vi "FGV_PSP - VRM Status.vi"(4 "error in":errorcluster, 6 "Function":enum16{"write", "read"}(ring), 7 "VRM status":T1={"X Target (T)"=0.0, "Y Target (T)"=0.0, "Z Target (T)"=0.0, "X Field (T)"=-0.0, "Y Field (T)"=0.0, "Z Field (T)"=0.0, "X Rate (T/min)"=0.0002, "Y Rate (T/min)"=0.0002, "Z Rate (T/min)"=0.05, "X Current (A)"=-0.0001, "Y Current (A)"=0.0001, "Z Current (A)"=0.0, "X Voltage (V)"=0.0003, "Y Voltage (V)"=0.0, "Z Voltage (V)"=-0.0001}) -> (0 "error out":errorcluster, 3 "VRM status":T1)   [LabVIEW 2016]
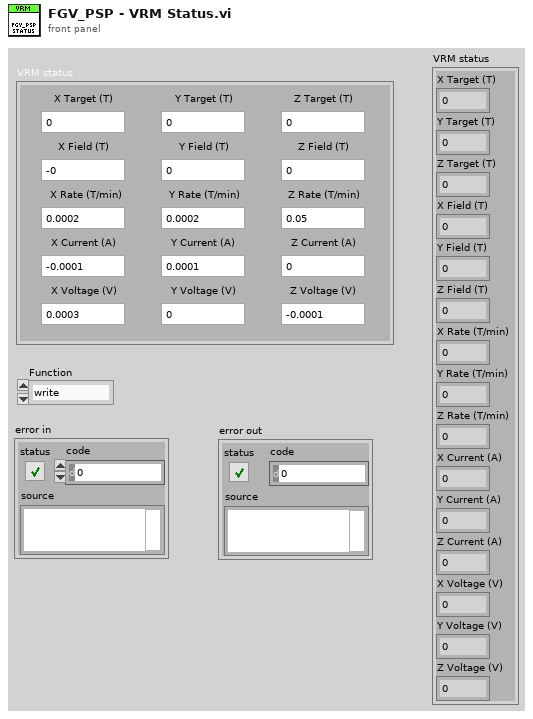
[diagram p1: front panel]
types:
  T1 = cluster{"X Target (T)":dbl, "Y Target (T)":dbl, "Z Target (T)":dbl, "X Field (T)":dbl, "Y Field (T)":dbl, "Z Field (T)":dbl, "X Rate (T/min)":dbl, "Y Rate (T/min)":dbl, "Z Rate (T/min)":dbl, "X Current (A)":dbl, "Y Current (A)":dbl, "Z Current (A)":dbl, "X Voltage (V)":dbl, "Y Voltage (V)":dbl, "Z Voltage (V)":dbl}
  T2 = cluster{"[0]":dbl, "[1]":dbl, "[2]":dbl, "[3]":dbl, "[4]":dbl, "[5]":dbl, "[6]":dbl, "[7]":dbl, "[8]":dbl, "[9]":dbl, "[10]":dbl, "[11]":dbl, "[12]":dbl, "[13]":dbl, "[14]":dbl}
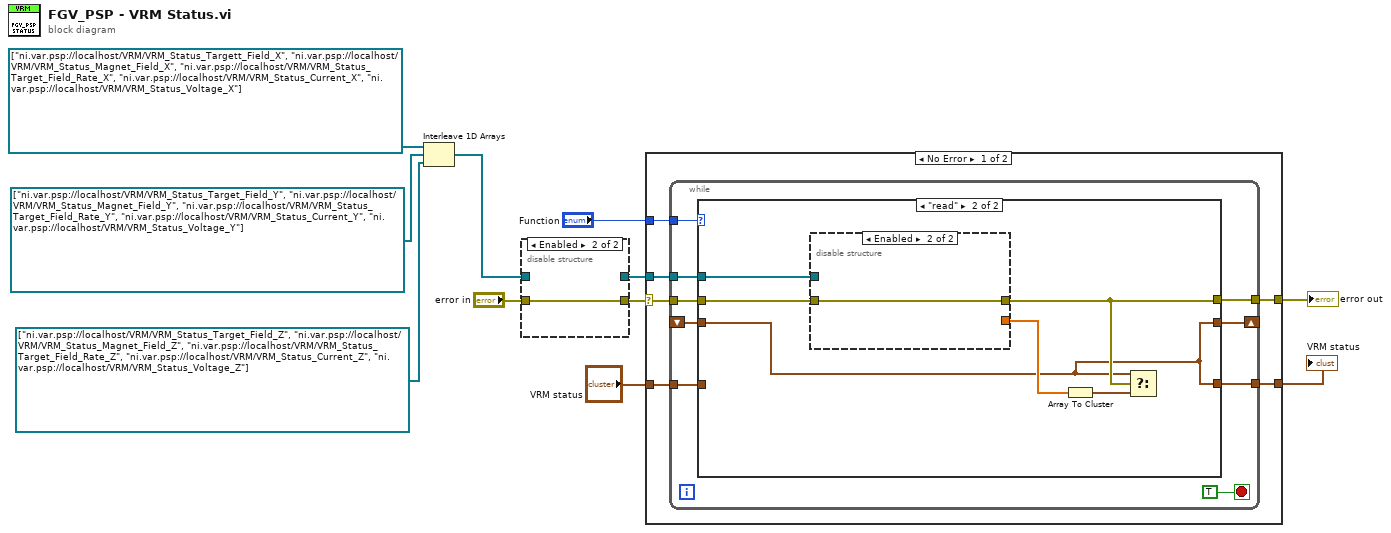
[diagram p0: block diagram]
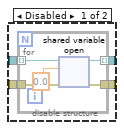
[diagram p2: hidden frame]
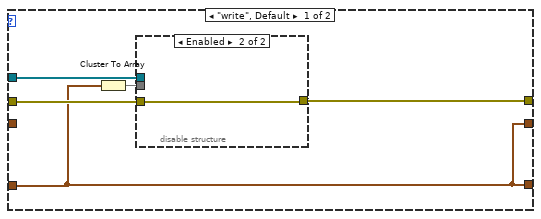
[diagram p3: hidden frame]
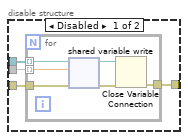
[diagram p4: hidden frame]
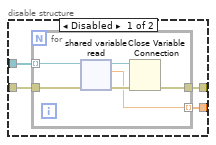
[diagram p5: hidden frame]
diagram:
  n1 = Interleave 1D Arrays(refnum<k21>[] ["ni.var.psp://localhost/VRM/VRM_Status_Targett_Field_X", "ni.var.psp://localhost/VRM/VRM_Status_Magnet_Field_X", "ni.var.psp://localhost/VRM/VRM_Status_Target_Field_Rate_X", "ni.var.psp://localhost/VRM/VRM_Status_Current_X", "ni.var.psp://localhost/VRM/VRM_Status_Voltage_X"], refnum<k21>[] ["ni.var.psp://localhost/VRM/VRM_Status_Target_Field_Y", "ni.var.psp://localhost/VRM/VRM_Status_Magnet_Field_Y", "ni.var.psp://localhost/VRM/VRM_Status_Target_Field_Rate_Y", "ni.var.psp://localhost/VRM/VRM_Status_Current_Y", "ni.var.psp://localhost/VRM/VRM_Status_Voltage_Y"], refnum<k21>[] ["ni.var.psp://localhost/VRM/VRM_Status_Target_Field_Z", "ni.var.psp://localhost/VRM/VRM_Status_Magnet_Field_Z", "ni.var.psp://localhost/VRM/VRM_Status_Target_Field_Rate_Z", "ni.var.psp://localhost/VRM/VRM_Status_Current_Z", "ni.var.psp://localhost/VRM/VRM_Status_Voltage_Z"]) -> (w1:refnum<k21>[])
  n2 = disable-structure shown="Enabled" {
    disable-tunnel: "error in" -> [w15 w21]
    disable-tunnel: [w14 _] -> w7
    disable-tunnel: [w13 w21] -> w5
    disable-tunnel: w1 -> [w12 _]
    frame Disabled {
      n3 = for {
        tunnel: w12 -> [w20] mode=indexing
        tunnel: [w18] -> w14 mode=indexing
        tunnel: [w17] -> w13
        tunnel: w15 -> [w16]
        n4 = shared-variable-open(w20, w16, 0.0) -> (w18:refnum<k21>, w17:errorcluster)  [unwired: 1 in]
      }
    }
    frame Enabled {
    }
  }
  n5 = case shown="No Error" w5 {
    selector: w5 -> [w27 w71]
    tunnel: [w26 w71] -> w11
    tunnel: "VRM status" -> [w25 w70]
    tunnel: [w24 w70] -> w9
    tunnel: "Function" -> [w23 _]
    tunnel: w7 -> [w22 _]
    frame No Error {
      n6 = while {
        shift-right: [w30] -> _
        shift-left: _ -> [w29]
        tunnel: w27 -> [w35]
        tunnel: [w34] -> w26
        tunnel: w25 -> [w33]
        tunnel: [w32] -> w24
        tunnel: w23 -> [w31]
        tunnel: w22 -> [w28]
        stop <- TRUE stop-if-true
        n7 = case shown="\"read\"" w31 {
          tunnel: w35 -> [w40 w58]
          tunnel: [w37 w57] -> w34
          tunnel: w33 -> [w39 _]
          tunnel: [w39 w53] -> w32
          tunnel: [w39 w53] -> w30
          tunnel: w29 -> [_ w53]
          tunnel: w28 -> [w41 w55]
          frame "write", Default {
            n8 = Cluster To Array(cluster=w39) -> (array=w38:dbl[])
            n9 = disable-structure shown="Enabled" {
              disable-tunnel: w41 -> [w45 _]
              disable-tunnel: w40 -> [w44 w52]
              disable-tunnel: w38 -> [w43 _]
              disable-tunnel: [w42 w52] -> w37
              frame Disabled {
                n10 = for {
                  tunnel: w44 -> [w51]
                  tunnel: w45 -> [w48] mode=indexing
                  tunnel: w43 -> [w47] mode=indexing
                  tunnel: [w46] -> w42
                  n11 = shared-variable-write(w48, w51, w47) -> (w49:refnum<k21>, w50:errorcluster)
                  n12 = Close Variable Connection(8:w50, 11:w49) -> (0:w46:errorcluster)
                }
              }
              frame Enabled {
              }
            }
          }
          frame "read" {
            n13 = disable-structure shown="Enabled" {
              disable-tunnel: w58 -> [w62 w69]
              disable-tunnel: [w61 w69] -> w57
              disable-tunnel: [w60 _] -> w56
              disable-tunnel: w55 -> [w59 _]
              frame Disabled {
                n14 = for {
                  tunnel: [w65] -> w60 mode=indexing
                  tunnel: [w66] -> w61
                  tunnel: w62 -> [w64]
                  tunnel: w59 -> [w63] mode=indexing
                  n15 = shared-variable-read(w63, w64) -> (w68:refnum<k21>, w67:errorcluster, w65:dbl)  [unwired: 1 out]
                  n16 = Close Variable Connection(8:w67, 11:w68) -> (0:w66:errorcluster)
                }
              }
              frame Enabled {
              }
            }
            n17 = Array To Cluster(array=w56) -> (cluster=w54:T2)
            n18 = Select(t=w53, s=w57, f=w54) -> ()  [unwired: 1 out]
          }
        }
      }
    }
    frame Error {
    }
  }
  "error out" <- w11
  "VRM status" <- w9
